vi "HiTechnic IRSeeker Sensor_AC_all_DM.vi"(2 "NXT/EV3":T4, 3 "Port/MUX":T2 {"Port" items=["Port 1", "Port 2", "Port 3", "Port 4"]; "MUX Port" items=["No MUX", "MUX 1", "MUX 2", "MUX 3", "MUX 4"]}) -> (0 "Success?":bool, 1 "All Info":T1, 4 "NXT/EV3":T4)   [LabVIEW 2012]
doc: "Reads the HiTechnic IRSeeker V2 Sensor in AC mode connected to the specified port and outputs a cluster containing the direction value as well an array of signal strengths from the five internal IR sensor elements. The direction value is in the range of 0 to 9 with 0 representing no IR detected; 1 to 9 represents a direction in a CW semi-circle around the sensor of which 5 indicates the IR source is straight ahead. In AC mode the sensor concentrates on a pulsating signal of either 600Hz or 1200Hz depending on the configuration setting.\n\n<B>Inputs\nNXT/EV3 </B> connects to NXT/EV3 terminal of previous VI to establish the flow of the program.\n<B>Port/MUX </B> is the port used for the sensor. This is a cluster that consists of the NXT/EV3 port as well as the HiTechnic Sensor Multiplexer (MUX) port. If the MUX is not used, then set this field to <B>No MUX</B>.\n\n<B>Outputs\nNXT/EV3 </B> wires to NXT/EV3 terminal of next VI to establish the flow of the program.\n<B>All Info </B> is a cluster containing the direction value as well as a 5 element array of signal strengths."
uses:
  <vilib>/NXT/Subs/LVHSConnector.ctl
  <vilib>/NXT/LegoClasses/BrickReference/BrickReference.lvclass
  <vilib>/NXT/HiTechnic/HiTechnic Controls/HiTechnic Port.ctl
  <vilib>/NXT/Block Support/NXT_InputPort.ctl
panel:
  # "HiTechnic IRSeeker Sensor VI\n\nThis VI reads the HiTechnic IRSeeker Sensor and \nreturns the current heading.\n\nFor more information go to www.hitechnic.com\nor email support@hitechnic.com\n(c) 2007 - 2009 HiTechnic"
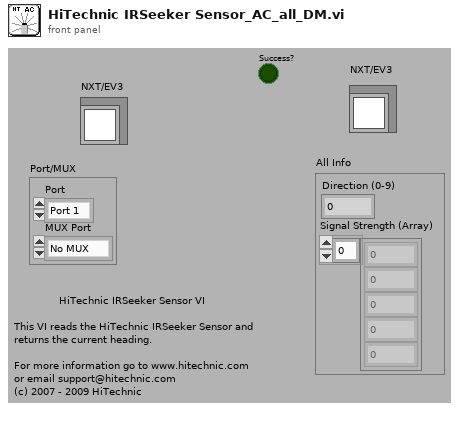
[diagram p1: front panel]
types:
  T1 = cluster{"Direction (0-9)":i16, "Signal Strength (Array)":u8[]}
  T2 = typedef "HiTechnic Port.ctl" = cluster{"Port":T3, "MUX Port":u8}
  T3 = typedef "NXT_InputPort.ctl" = u32
  T4 = typedef "LVHSConnector.ctl" = refnum<class "BrickReference.lvclass">
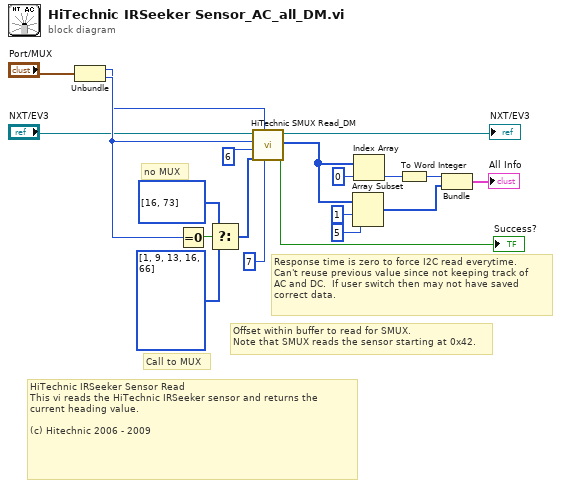
[diagram p0: block diagram]
diagram:
  # "Response time is zero to force I2C read everytime.\nCan't reuse previous value since not keeping track of\nAC and DC.  If user switch then may not have saved \ncorrect data."
  # "Offset within buffer to read for SMUX.  \nNote that SMUX reads the sensor starting at 0x42."
  # "no MUX"
  # "Call to MUX"
  # "HiTechnic IRSeeker Sensor Read\nThis vi reads the HiTechnic IRSeeker sensor and returns the\ncurrent heading value.  \n\n(c) Hitechnic 2006 - 2009"
  n1 = Unbundle("Port/MUX") -> ("Port"=w19:T3, "MUX Port"=w20:u8)
  n2 = Equal To 0?(x=w20) -> (x = 0?=w15:bool)
  n3 = Select(t=u8[] [16, 73] ("Buffer"), s=w15, f=u8[] [1, 9, 13, 16, 66]) -> (s? t:f=w18:u8[])
  n4 = call "HiTechnic SMUX Read_DM.vi"("Offset"=u8 7, "Port"=w19, "Parameters"=w18, "Read Length"=u8 6, "MUX Port"=w20, "NXT/EV3"="NXT/EV3") -> ("Success?"=→"Success?":bool, "Array"=w5:u8[], "NXT/EV3"=→"NXT/EV3":T4)  [unwired: 3 in]
  n5 = Array Subset(array=w5, index=1, length=5) -> (w6:u8[])
  n6 = Index Array(array=w5, index=0) -> (element=w3:u8)
  n7 = To Word Integer(number=w3) -> (16bit integer=w4:i16)
  n8 = Bundle(w4, w6) -> (→"All Info":cluster{i16, u8[]})  [unwired: 1 in]
